vi "_Read.vi"(8 "error in (no error)":errorcluster, 11 "Keithley Multimeter in":refnum<class "Testing Keithley Multimeter.lvclass">) -> (0 "error out":errorcluster, 2 "appended array":dbl[](array[numeric]), 3 "Keithley Multimeter out":refnum<class "Testing Keithley Multimeter.lvclass">)   [LabVIEW 2017, in "Testing Keithley Multimeter.lvclass"]
doc: "(Protected, Dynamic, Pure Virtual/Abstract) Perform a measurement and return one or more channels of data. Outsiders should not call this method, but instead the public \"Read Data.vi\"."
uses:
  Testing Keithley Multimeter.lvclass
  Testing Keithley Multimeter.lvclass/Testing Keithley Multimeter.ctl
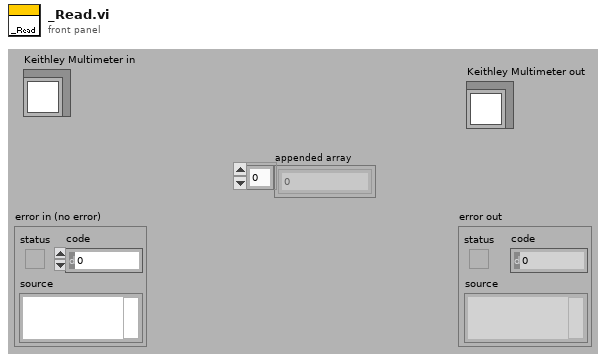
[diagram p1: front panel]
types:
  T1 = cluster{"error":bool, "code":i32, "source":string}
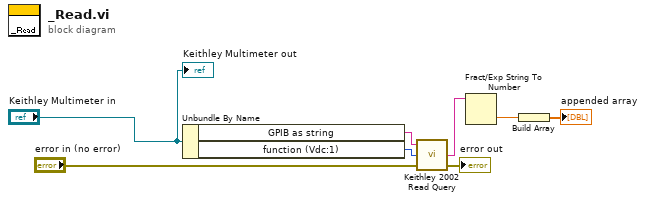
[diagram p0: block diagram]
diagram:
  n1 = Unbundle By Name("Keithley Multimeter in") -> ("GPIB as string"=w5:string, "function (Vdc:1)"=w6:u16)
  n2 = call "Keithley 2002 Read Query.vi"("error in"="error in (no error)", "function (Vdc:1)"=w6, "GPIB Address"=w5) -> ("error out"=→"error out":T1, "Reading Result"=w8:string)  [unwired: 1 in]
  n3 = Fract/Exp String To Number(string=w8) -> (number=w4:dbl)  [unwired: 3 in, 1 out]
  n4 = Build Array(w4) -> (→"appended array":dbl[])
  "Keithley Multimeter out" <- "Keithley Multimeter in"
